vi "GetCtrlRefInCluster.vi"(8 "error in (no error)":errorcluster caption="エラー入力（エラーなし）", 10 "Ctl name":string, 11 "clust ref":refnum<vi>) -> (0 "error out":errorcluster caption="エラー出力", 3 "Ctl refnum":refnum<vi>)   [LabVIEW 2016]
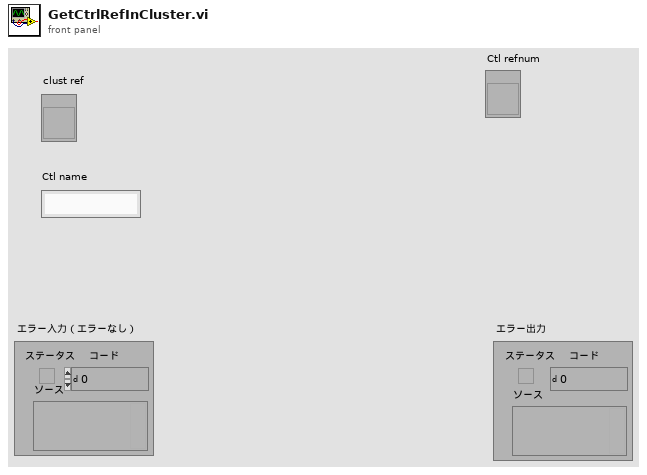
[diagram p1: front panel]
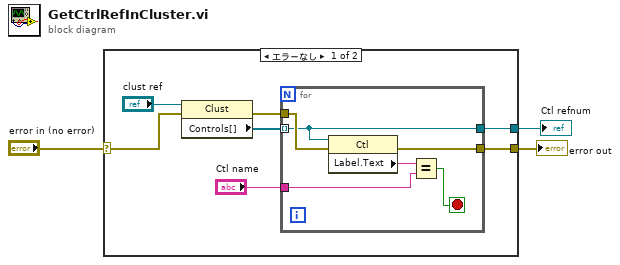
[diagram p0: block diagram]
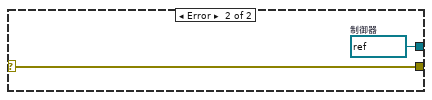
[diagram p2: hidden frame]
diagram:
  n1 = case shown="エラーなし" "error in (no error)" {
    selector: "error in (no error)" -> [w9 w18]
    tunnel: [w5 w18] -> w2
    tunnel: [w4 w17] -> w1
    frame No Error {
      n2 = property class="Clust"(reference="clust ref", error in=w9) -> (error out=w7:errorcluster, "Controls[]"=w8:refnum<vi>[])  [unwired: 1 out]
      n3 = for {
        tunnel: w8 -> [w13] mode=indexing
        tunnel: w7 -> [w16]
        tunnel: "Ctl name" -> [w14]
        tunnel: [w13] -> w4
        tunnel: [w11] -> w5
        stop <- w12 stop-if-true
        n4 = property class="Ctl"(reference=w13, error in=w16) -> (error out=w11:errorcluster, "Label.Text"=w15:string)  [unwired: 1 out]
        n5 = Equal?(x=w15, y=w14) -> (x = y?=w12:bool)
      }
    }
    frame Error {
      w17 = refnum<vi> refnum  # 制御器
    }
  }
  "error out" <- w2
  "Ctl refnum" <- w1
